vi "Reorder Functions on Priority.vi"(0 "config path":path, 5 "Function List":string[](array[string]), 11 "error in (no error)":errorcluster) -> (6 "Function List out":string[](array[string]), 15 "error out":errorcluster)   [LabVIEW 2019, in "LSL.lvlib" / "scripts manager.lvclass"]
uses:
  scripts manager.lvclass
  <vilib>/Utility/config.llb/Read Key (Boolean).vi
  <vilib>/Utility/config.llb/NI_LVConfig.lvlib
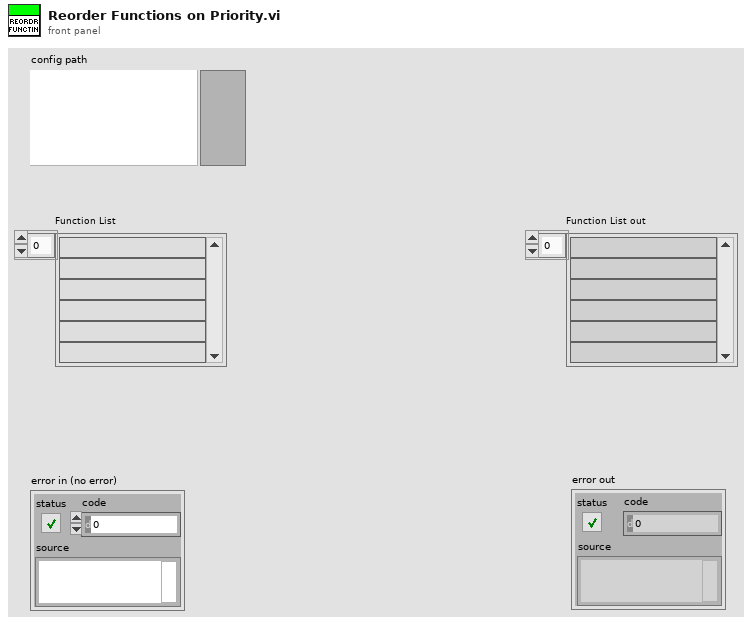
[diagram p1: front panel]
types:
  T1 = typedef "NI_LVConfig.lvlib/Config Data RefNum.ctl" = refnum<k1>
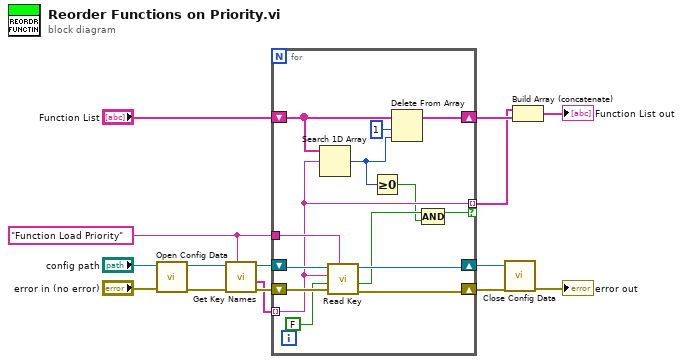
[diagram p0: block diagram]
diagram:
  w8 = "Function Load Priority" ("section")
  n1 = call <vilib>:"Open Config Data.vi"("error in (no error)"="error in (no error)", "configuration file path"="config path") -> ("error out"=w12:errorcluster, "refnum"=w13:T1)  [unwired: 7 in, 1 out]
  n2 = call <vilib>:"Get Key Names.vi"("section"=w8, "error in (no error)"=w12, "refnum"=w13) -> ("error out"=w11:errorcluster, "key names"=w9:string[], "refnum out"=w10:T1)  [unwired: 5 in, 1 out]
  n3 = for {
    shift-right: [w25] -> w6
    shift-left: w10 -> [w29]
    shift-right: [w26] -> w7
    shift-left: w11 -> [w28]
    tunnel: w9 -> [w20] mode=indexing
    tunnel: w8 -> [w24]
    shift-right: [w22] -> w3
    shift-left: "Function List" -> [w23]
    tunnel: [w20] -> w2 mode=indexing if=w17
    n4 = Search 1D Array(1D array=w23, element=w20) -> (index of element=w18:i32)  [unwired: 1 in]
    n5 = call-poly <vilib>:"Read Key.vi"("section"=w24, "error in (no error)"=w28, "default value"=FALSE, "key"=w20, "refnum"=w29) -> ("error out"=w26:errorcluster, "value"=w19:bool, "refnum out"=w25:T1)  [unwired: 3 in, 1 out]
    n6 = Greater Or Equal To 0?(x=w18) -> (x >= 0?=w16:bool)
    n7 = Delete From Array(array=w23, length=1, index=w18) -> (array with subset deleted=w22:string[])  [unwired: 1 out]
    n8 = Compound Arithmetic op=AND(w19, w16) -> (w17:bool)
  }
  n9 = call <vilib>:"Close Config Data.vi"("error in (no error)"=w7, "refnum"=w6) -> ("error out"=→"error out":errorcluster)  [unwired: 8 in, 1 out]
  n10 = Build Array (concatenate)(w2, w3) -> (→"Function List out":string[])
